vi "Sub_ shift data reset.vi"(8 "Serial no":string="Counter.txt", 9 "Shift":string, 10 "Model":string) -> (1 "Serial no":string, 2 "Barcode data":string[](array[string]))   [LabVIEW 2015]
uses:
  <vilib>/Utility/file.llb/Read Delimited Spreadsheet (string).vi
panel:
  out "appended path":path
  out "Serch index":i32
  out "subarray":string[](array[string])
  out "date string":string
  out "data":string[][](table)
  out "error out":errorcluster
  out "Serial No":i32
  # "Barcode information"
  # "Date"
  # "Shift"
  # "Model Name"
  # "Company name"
  # "Barcode"
  # "PartName"
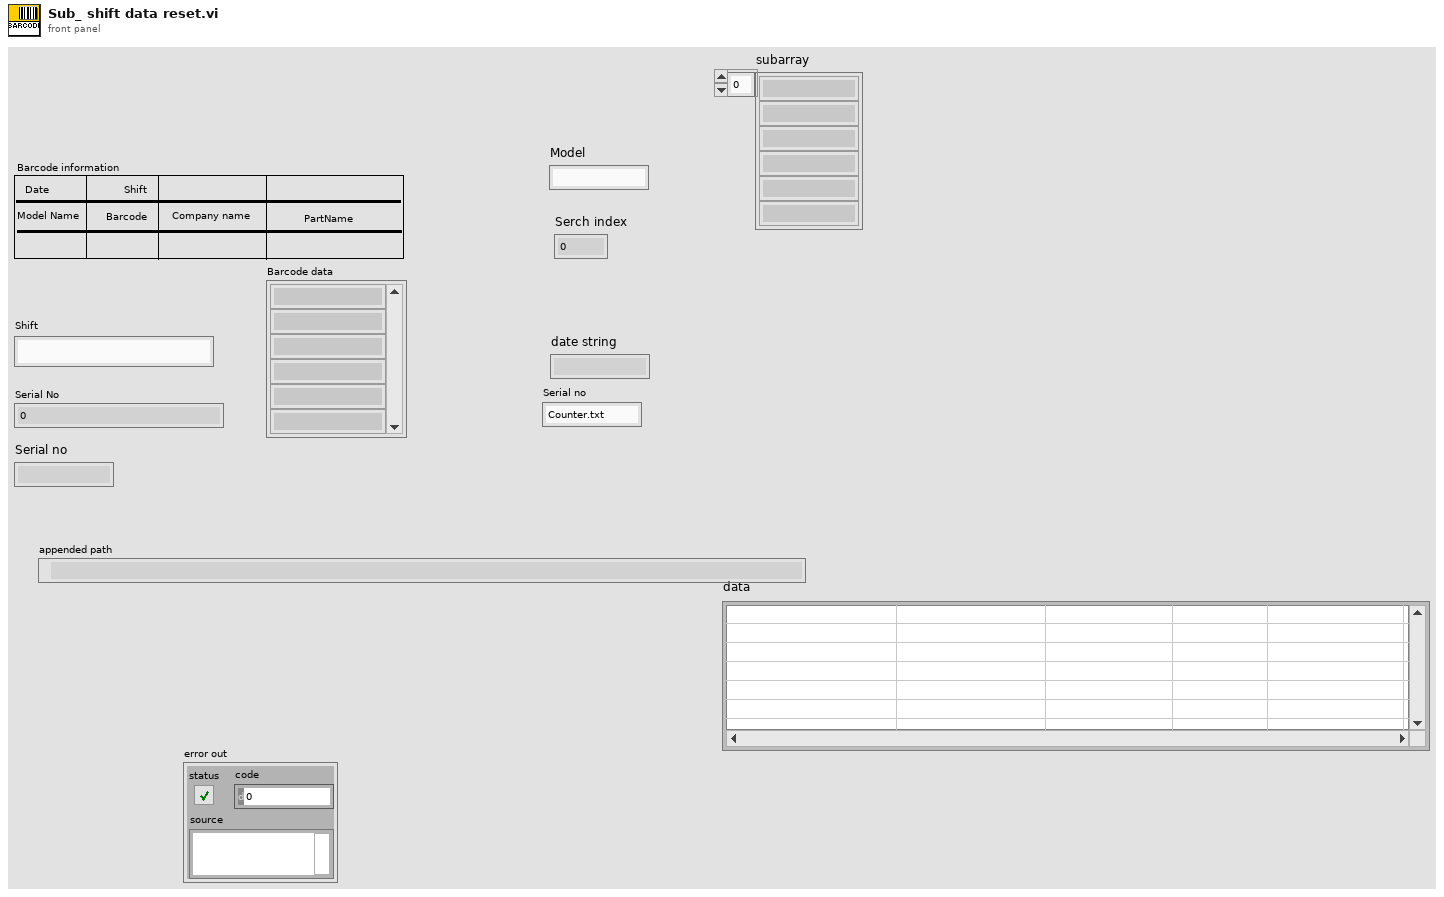
[diagram p1: front panel]
types:
  T1 = enum16{"open", "replace", "create", "open or create", "replace or create", "replace or create with confirmation"}
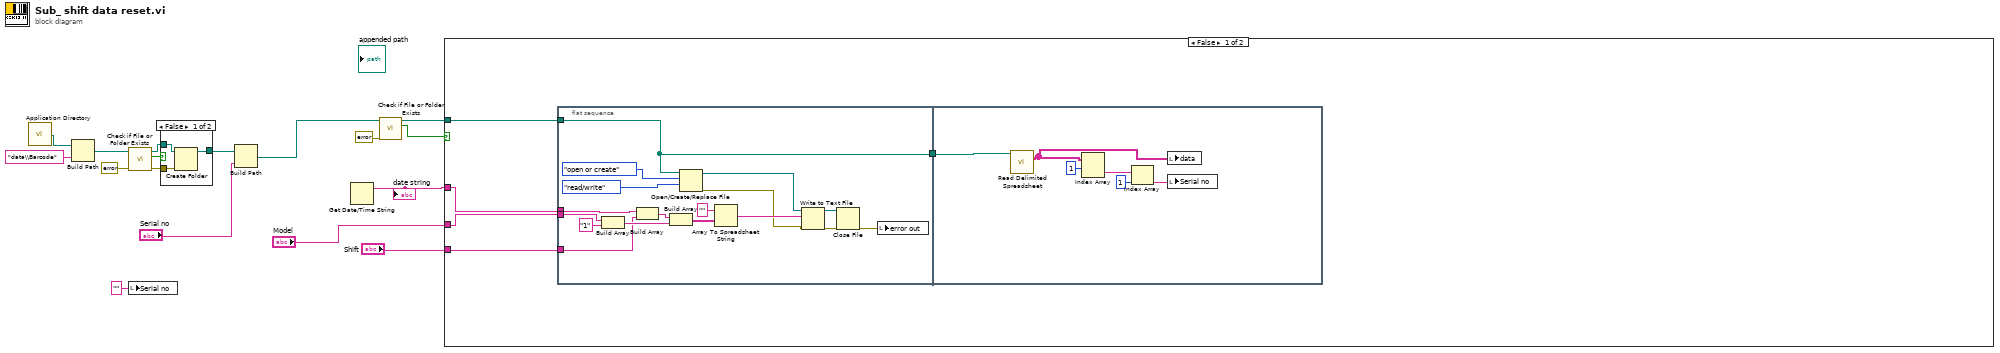
[diagram p0: block diagram]
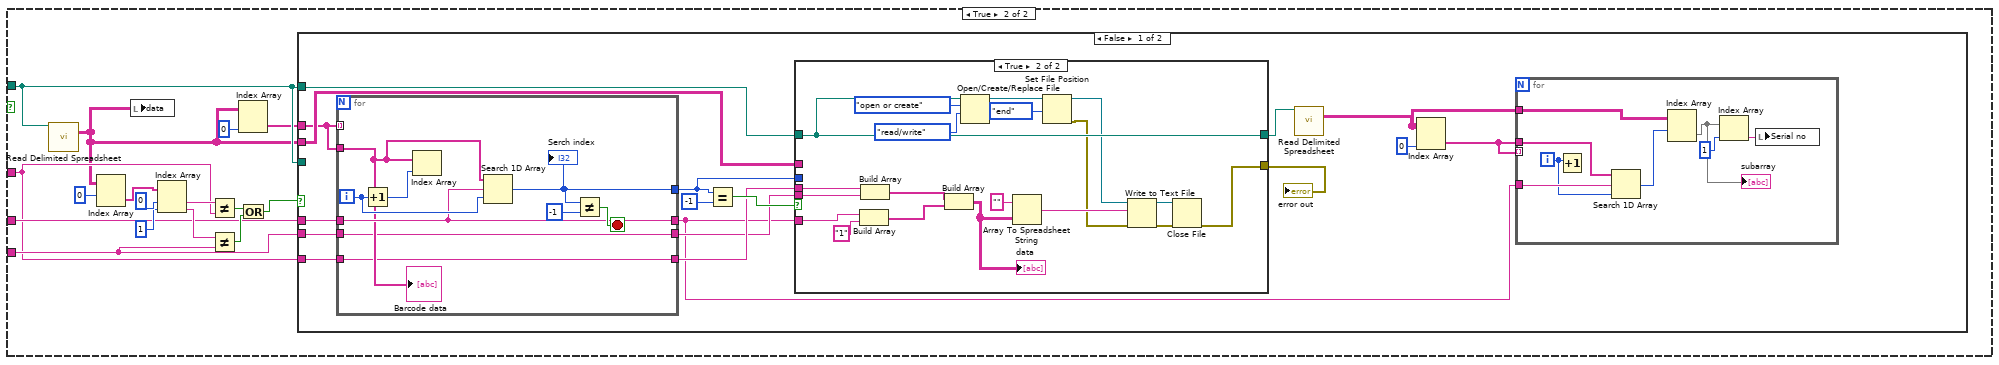
[diagram p3: hidden frame]
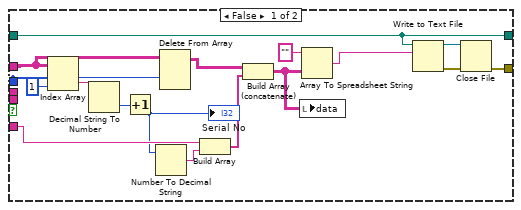
[diagram p4: hidden frame]
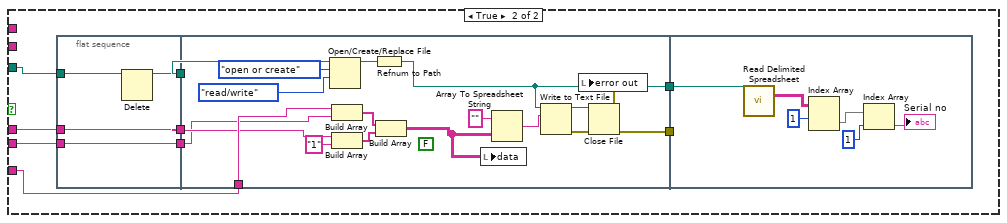
[diagram p5: hidden frame]
diagram:
  n1 = call <vilib>:"Application Directory.vi"() -> ("Application Directory"=w11:path)
  n2 = Build Path(base path=w11, name or relative path="data\\Barcode") -> (appended path=w9:path)
  n3 = local write "Serial no"("" ("Serial no")) -> ()
  n4 = call <vilib>:"Check if File or Folder Exists.vi"("error in (no error)"=errorcluster {"status"=FALSE, "code"=0, "source"=""}, "path"=w9) -> ("error out"=w8:errorcluster, "file or folder exists?"=w6:bool, "dup path"=w10:path)  [unwired: 7 in]
  n5 = case shown="False" w6 {
    tunnel: w10 -> [w20 w21]
    tunnel: [w19 w21] -> w5
    tunnel: w8 -> [w18 _]
    frame False {
      n6 = Create Folder(path (use dialog)=w20, error in=w18) -> (created path=w19:path)  [unwired: 1 in, 2 out]
    }
    frame True {
    }
  }
  n7 = Build Path(base path=w5, name or relative path="Serial no") -> (appended path=w3:path)
  n8 = Get Date/Time String() -> (date string=w13:string)  [unwired: 3 in, 1 out]
  "date string" <- w13
  n9 = call <vilib>:"Check if File or Folder Exists.vi"("error in (no error)"=errorcluster {"status"=FALSE, "code"=0, "source"=""}, "path"=w3) -> ("file or folder exists?"=w15:bool, "dup path"=w17:path)  [unwired: 7 in, 1 out]
  n10 = case shown="False" w15 {
    tunnel: w17 -> [w23 w53]
    tunnel: w13 -> [w26 w54]
    tunnel: "Shift" -> [w25 w55]
    tunnel: "Model" -> [w24 w56]
    frame False {
      n11 = flat-sequence {
        tunnel: w26 -> [w38]
        tunnel: w25 -> [w37]
        tunnel: w24 -> [w36]
        tunnel: w23 -> [w29]
        tunnel: [w29] -> w22
        tunnel: w22 -> [w49]
        frame #0 {
          n12 = Build Array(w36, "1" ("element")) -> (w39:string[])
          n13 = Build Array(w38, w37) -> (w40:string[])
          n14 = Build Array(w40, w39) -> (w32:string[][])
          n15 = Open/Create/Replace File(file path (use dialog)=w29, operation (0:open)=T1."open or create", access (0:read/write)=enum16{"read/write", "read-only", "write-only"}."read/write") -> (refnum out=w28:refnum<file>, error out=w27:errorcluster)  [unwired: 3 in, 1 out]
          n16 = Array To Spreadsheet String(array=w32, 3:"" ("format string")) -> (spreadsheet string=w34:string)  [unwired: 1 in]
          n17 = Write to Text File(file (use dialog)=w28, text=w34, error in=w27) -> (refnum out=w33:refnum<file>, error out=w35:errorcluster)  [unwired: 1 in, 1 out]
          n18 = Close File(refnum=w33, error in=w35) -> (error out=w30:errorcluster)  [unwired: 1 out]
          n19 = local write "error out"(w30) -> ()
        }
        frame #1 {
          n20 = call-poly <vilib>:"Read Delimited Spreadsheet.vi"("file path (dialog if empty)"=w49) -> ("all rows"=w44:string[][])  [unwired: 9 in, 5 out]
          n21 = Index Array(array=w44, index (row)=1) -> (element=w47:string[])  [unwired: 1 in]
          n22 = Index Array(array=w47, index=1) -> (element=w45:string)
          n23 = local write "data"(w44) -> ()
          n24 = local write "Serial no"(w45) -> ()
        }
      }
    }
    frame True {
      n25 = call-poly <vilib>:"Read Delimited Spreadsheet.vi"("file path (dialog if empty)"=w53) -> ("all rows"=w50:string[][])  [unwired: 9 in, 5 out]
      n26 = Index Array(array=w50, index (row)=0) -> (element=w64:string[])  [unwired: 1 in]
      n27 = local write "data"(w50) -> ()
      n28 = Index Array(array=w64, index #1=0 ("index"), index #2=1 ("index")) -> (element #1=w61:string, element #2=w60:string)
      n29 = Not Equal?(x=w61, y=w54) -> (x != y?=w59:bool)
      n30 = Not Equal?(x=w60, y=w55) -> (x != y?=w58:bool)
      n31 = Index Array(array=w50, index (col)=0 ("disabled index (col)")) -> (element=w51:string[])  [unwired: 1 in]
      n32 = Or(x=w59, y=w58) -> (x .or. y?=w57:bool)
      n33 = case shown="False" w57 {
        tunnel: w53 -> [_ w144]
        tunnel: w56 -> [w82 w141]
        tunnel: w55 -> [w71 w140]
        tunnel: w54 -> [w73 w138]
        tunnel: w50 -> [w77 _]
        tunnel: w53 -> [w79 _]
        tunnel: w51 -> [w76 _]
        frame False {
          n34 = for {
            tunnel: w82 -> [w130]
            tunnel: [w131] -> w78
            tunnel: [w130] -> w67
            tunnel: w76 -> [_] mode=indexing
            tunnel: w76 -> [w129]
            tunnel: [w128] -> w72
            tunnel: w73 -> [w128]
            tunnel: [w127] -> w70
            tunnel: w71 -> [w127]
            i -> [w133]
            stop <- w132 stop-if-true
            n35 = Increment(x=w133) -> (x+1=w135:i32)
            n36 = Index Array(array=w129, index=w135) -> ()  [unwired: 1 out]
            n37 = Search 1D Array(1D array=w129, element=w130, start index (0)=w133) -> (index of element=w131:i32)
            "Serch index" <- w131
            n38 = Not Equal?(x=w131, y=-1) -> (x != y?=w132:bool)
            "Barcode data" <- w129
          }
          n39 = Equal?(x=w78, y=-1) -> (x = y?=w80:bool)
          n40 = case shown="True" w80 {
            tunnel: w79 -> [w91 w112]
            tunnel: w67 -> [w101 w126]
            tunnel: w78 -> [w103 _]
            tunnel: w77 -> [w104 _]
            tunnel: [w94 w121] -> w75
            tunnel: [w91 w112] -> w74
            tunnel: w72 -> [_ w119]
            tunnel: w70 -> [_ w118]
            frame False {
              n41 = Index Array(array=w104, index (row)=w103, index (col)=1 ("disabled index (col)")) -> (element=w106:string)
              n42 = Decimal String To Number(string=w106) -> (number=w105:i32)  [unwired: 2 in, 1 out]
              n43 = Increment(x=w105) -> (x+1=w100:i32)
              "Serial No" <- w100
              n44 = Number To Decimal String(number=w100) -> (decimal integer string=w99:string)  [unwired: 1 in]
              n45 = Delete From Array(array=w104, index (row)=w103) -> (array with subset deleted=w102:string[][])  [unwired: 2 in, 1 out]
              n46 = Build Array(w101, w99) -> (w98:string[])
              n47 = Build Array (concatenate)(w102, w98) -> (w92:string[][])
              n48 = local write "data"(w92) -> ()
              n49 = Array To Spreadsheet String(array=w92, 3:"" ("format string")) -> (spreadsheet string=w97:string)  [unwired: 1 in]
              n50 = Write to Text File(file (use dialog)=w91, text=w97) -> (refnum out=w96:refnum<file>, error out=w95:errorcluster)  [unwired: 2 in, 1 out]
              n51 = Close File(refnum=w96, error in=w95) -> (error out=w94:errorcluster)  [unwired: 1 out]
            }
            frame True {
              n52 = Build Array(w126, "1" ("element")) -> (w116:string[])
              n53 = Build Array(w119, w118) -> (w117:string[])
              n54 = Build Array(w117, w116) -> (w115:string[][])
              "data" <- w115
              n55 = Open/Create/Replace File(file path (use dialog)=w112, operation (0:open)=T1."open or create", access (0:read/write)=enum16{"read/write", "read-only", "write-only"}."read/write") -> (refnum out=w111:refnum<file>)  [unwired: 3 in, 2 out]
              n56 = Array To Spreadsheet String(array=w115, 3:"" ("format string")) -> (spreadsheet string=w123:string)  [unwired: 1 in]
              n57 = Set File Position(refnum=w111, from (0:start)=enum16{"start", "end", "current"}."end") -> (refnum out=w109:refnum<file>, error out=w108:errorcluster)  [unwired: 2 in]
              n58 = Write to Text File(file (use dialog)=w109, text=w123, error in=w108) -> (refnum out=w122:refnum<file>, error out=w124:errorcluster)  [unwired: 1 in, 1 out]
              n59 = Close File(refnum=w122, error in=w124) -> (error out=w121:errorcluster)  [unwired: 1 out]
            }
          }
          "error out" <- w75
          n60 = call-poly <vilib>:"Read Delimited Spreadsheet.vi"("file path (dialog if empty)"=w74) -> ("all rows"=w66:string[][])  [unwired: 9 in, 5 out]
          n61 = Index Array(array=w66, index (col)=0 ("disabled index (col)")) -> (element=w68:string[])  [unwired: 1 in]
          n62 = for {
            tunnel: w66 -> [w85]
            tunnel: w68 -> [w87]
            tunnel: w68 -> [_] mode=indexing
            tunnel: w67 -> [w88]
            i -> [w86]
            n63 = Increment(x=w86) -> ()  [unwired: 1 out]
            n64 = Search 1D Array(1D array=w87, element=w88, start index (0)=w86) -> (index of element=w84:i32)
            n65 = Index Array(array=w85, index (row)=w84) -> (element=w83:string[])  [unwired: 1 in]
            "subarray" <- w83
            n66 = Index Array(array=w83, index=1) -> (element=w89:string)
            n67 = local write "Serial no"(w89) -> ()
          }
        }
        frame True {
          n68 = flat-sequence {
            tunnel: w144 -> [w146]
            tunnel: [w145] -> w143
            tunnel: [w148] -> w142
            tunnel: w141 -> [w148]
            tunnel: w140 -> [w147]
            tunnel: [w147] -> w139
            tunnel: w143 -> [w164]
            tunnel: w142 -> [w160]
            tunnel: w139 -> [w149]
            tunnel: w138 -> [w161]
            tunnel: [w151] -> w137
            tunnel: [w152] -> w136
            tunnel: w137 -> [_]
            tunnel: w136 -> [w171]
            frame #0 {
              n69 = Delete(path (use dialog)=w146) -> (deleted path=w145:path)  [unwired: 4 in, 2 out]
            }
            frame #1 {
              (unwired) FALSE ("append to file? (new file:F)")
              n70 = Open/Create/Replace File(file path (use dialog)=w164, operation (0:open)=T1."open or create", access (0:read/write)=enum16{"read/write", "read-only", "write-only"}."read/write") -> (refnum out=w165:refnum<file>)  [unwired: 3 in, 2 out]
              n71 = Build Array(w161, w149) -> (w158:string[])
              n72 = Build Array(w160, "1" ("element")) -> (w157:string[])
              n73 = Refnum to Path(1:w165) -> (0:w152:path)
              n74 = Build Array(w158, w157) -> (w150:string[][])
              n75 = local write "data"(w150) -> ()
              n76 = Array To Spreadsheet String(array=w150, 3:"" ("format string")) -> (spreadsheet string=w155:string)  [unwired: 1 in]
              n77 = Write to Text File(file (use dialog)=w152, text=w155) -> (refnum out=w154:refnum<file>, error out=w156:errorcluster)  [unwired: 2 in, 1 out]
              n78 = Close File(refnum=w154, error in=w156) -> (error out=w151:errorcluster)  [unwired: 1 out]
              n79 = local write "error out"(w151) -> ()
            }
            frame #2 {
              n80 = call-poly <vilib>:"Read Delimited Spreadsheet.vi"("file path (dialog if empty)"=w171) -> ("all rows"=w166:string[][])  [unwired: 9 in, 5 out]
              n81 = Index Array(array=w166, index (row)=1) -> (element=w169:string[])  [unwired: 1 in]
              n82 = Index Array(array=w169, index=1) -> (element=→"Serial no":string)
            }
          }
        }
      }
    }
  }
